vi "Make Circle Rectangle.vi"(10 "Size":i32=3, 11 "Coordinate":cluster{dbl, dbl}) -> (3 "Rectangle":cluster{dbl, dbl, dbl, dbl})   [LabVIEW 2016]
doc: "This VI returns a bounding rectangle for a circle of a given size."
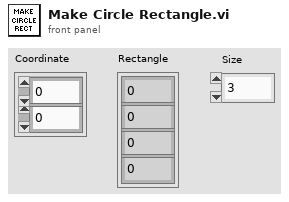
[diagram p1: front panel]
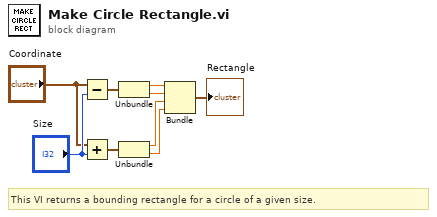
[diagram p0: block diagram]
diagram:
  # "This VI returns a bounding rectangle for a circle of a given size."
  n1 = Subtract(x="Coordinate", y="Size") -> (x-y=w9:cluster{dbl, dbl})
  n2 = Add(x="Coordinate", y="Size") -> (x+y=w8:cluster{dbl, dbl})
  n3 = Unbundle(w9) -> (w1:dbl, w3:dbl)
  n4 = Unbundle(w8) -> (w4:dbl, w5:dbl)
  n5 = Bundle(w1, w3, w4, w5) -> (→"Rectangle":cluster{dbl, dbl, dbl, dbl})  [unwired: 1 in]
